vi "HapticSPM_write_virtual_only.vi"() -> ()   [LabVIEW 2022 SP3]
uses:
  Haptic-Programming-Interface/LabVIEW VIs/Haptic Prog Interface/Haptic Prog Interface.lvlib
panel:
  out "Value":dbl caption="Numeric" format="%#_2p"
  in  "Stop":bool
  out "Force vs Signal":cluster{dbl[], dbl[]}(graph)
  out "Signal & Force (Scaled)":dbl[][](graph)
  in  "Suggested Settings":bool=TRUE
  out "?":bool=TRUE
  out "Surface":dbl caption="Numeric" format="%#_2p"
  out "Z-Position":dbl caption="Numeric" format="%#_2p"
  out "y":string
  out "x":string
  out "scan data":dbl[][](array[numeric])
  out "2D Picture":picture
  out "Force":dbl(slide) scale=-3.0..3.0
  out "Frame String":string
  out "Reframed Position (m)":cluster{"x (m)":dbl, "y (m)":dbl, "z (m)":dbl} {"z (m)" format="%.1p"; "y (m)" format="%.1p"; "x (m)" format="%.1p"}
  out "Frame Properties (m)":T1
  in  "Function":string(combo)="0" caption="Combo Box"
  in  "Gain (mm/pm)":dbl=1.0 caption="Numeric" format="%.1g"
  in  "k":dbl=1.0 caption="Numeric" step=0.1 format="%.1g"
  in  "Setpoint":dbl=1e-10 caption="Numeric" step=1e-11 format="%.0p"
  in  "Gain":dbl=1.0 caption="Numeric" format="%.1g"
  out "Click Number":dbl caption="Numeric" format="%#_1g"
  in  "Planing Toggle":bool
  in  "Planing Reset":bool
  in  "Save":bool
  # "Super Ultra Mega Haptic SPM Controller 3000"
  # "Scan Window"
  # "Height"
  # "Signal"
  # "Force"
  # "Force"
  # "Planing"
  # "Surface Scale"
  # "Move pens in all three dimensions to calibrate\nClick \"enter\" to turn off recommended settings"
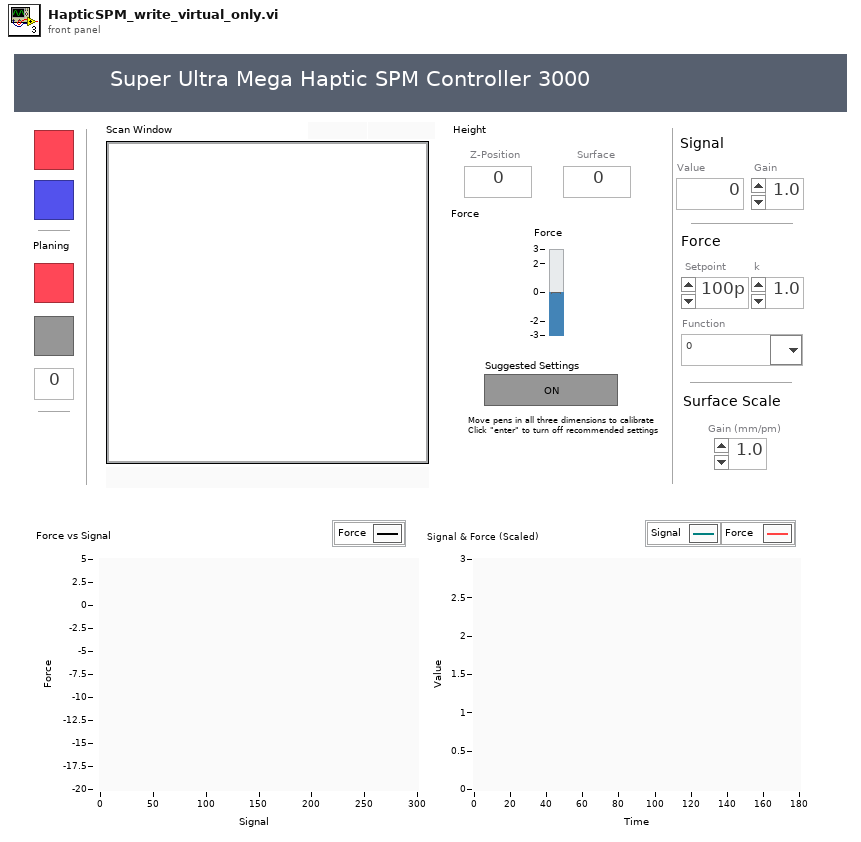
[diagram p1: front panel]
types:
  T1 = cluster{"Center coordinates (m)":cluster{"Xc":sgl, "Yc":sgl}, "Size (m)":cluster{"Width":sgl, "Height":sgl}}
  T2 = cluster{"Fx (N)":dbl, "Fy (N)":dbl, "Fz (N)":dbl}
  T3 = cluster{"kx (N/m)":dbl, "ky (N/m)":dbl, "kz (N/m)":dbl}
  T4 = cluster{"X Drag":bool, "Y Drag":bool, "Z Drag":bool}
  T5 = cluster{"Origin (m)":cluster{"X Origin (m)":dbl, "Y Origin (m)":dbl}, "Frame Size (m)":cluster{"FW (m)":dbl, "FH (m)":dbl}}
  T6 = cluster{"x (mm)":dbl, "y (mm)":dbl, "z (mm)":dbl}
  T7 = typedef "LVBoundsTypeDef.ctl" = cluster{"Width":u32, "Height":u32}
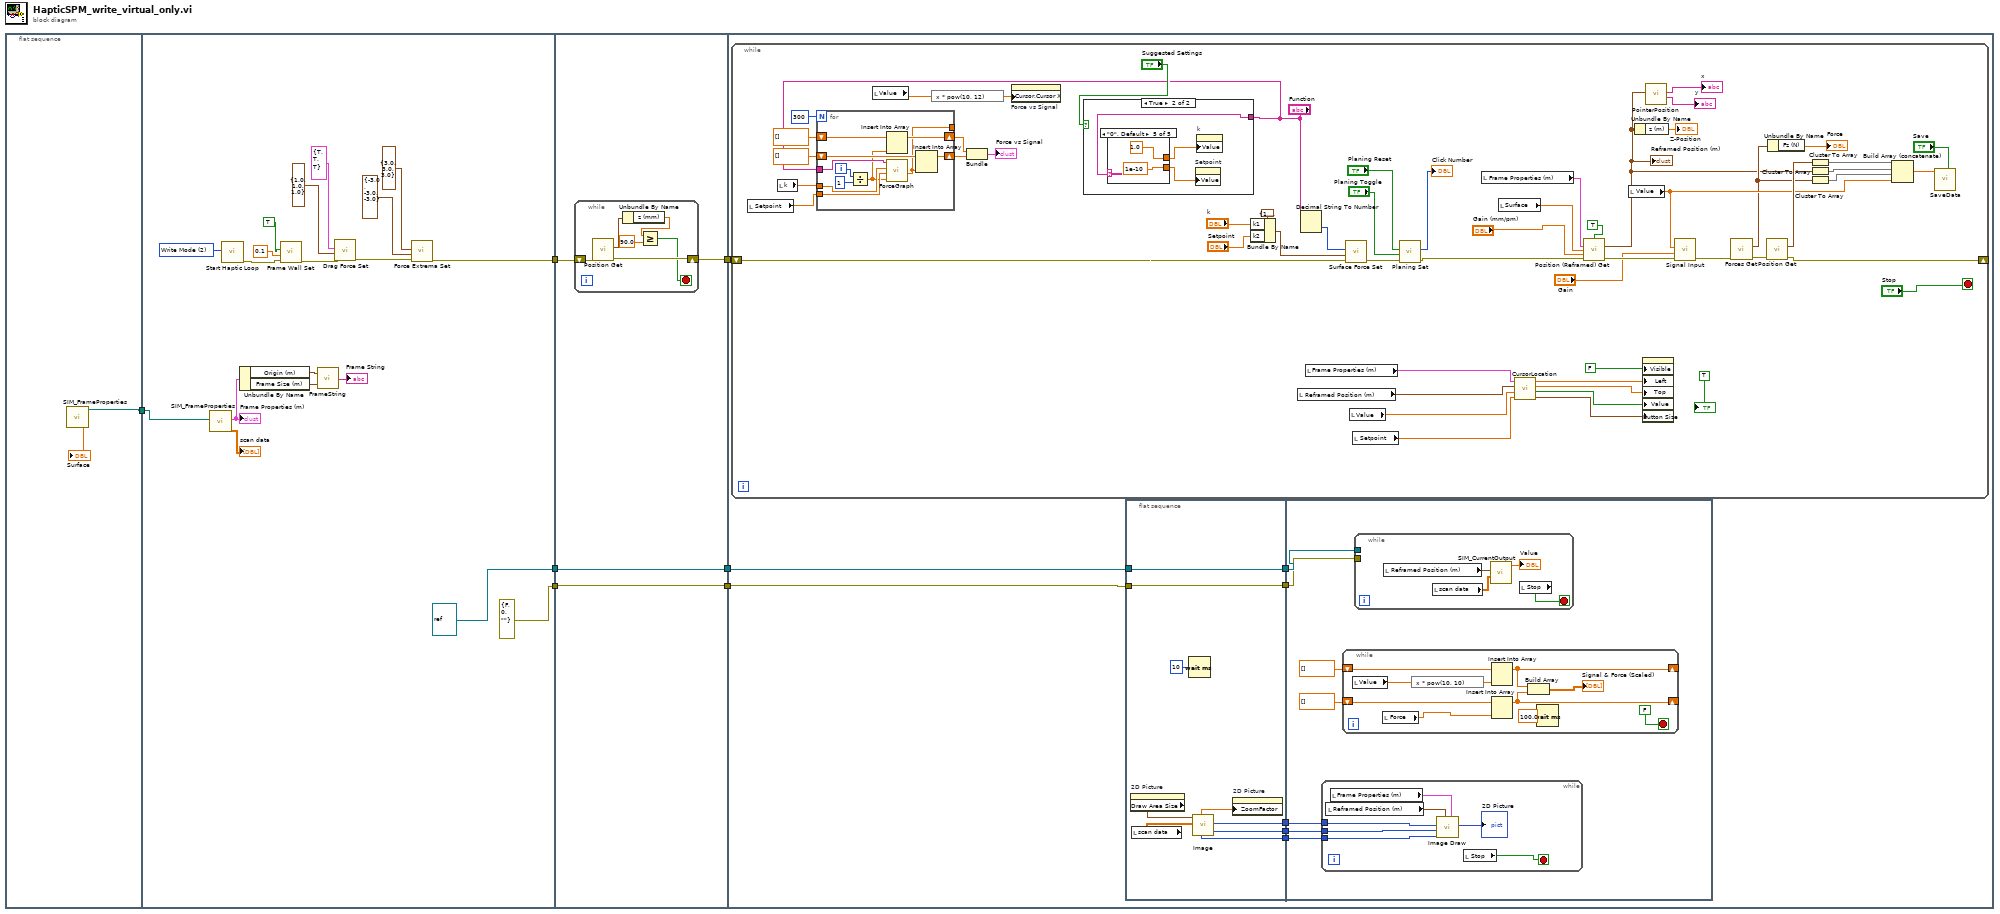
[diagram p0: block diagram]
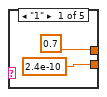
[diagram p3: hidden frame]
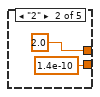
[diagram p4: hidden frame]
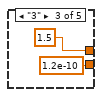
[diagram p5: hidden frame]
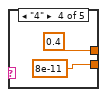
[diagram p6: hidden frame]
diagram:
  n1 = flat-sequence {
    tunnel: [w8] -> w1
    tunnel: [w26] -> w7
    tunnel: [refnum<vi> refnum ("Application ref out")] -> w4
    tunnel: [errorcluster {"status"=FALSE, "code"=0, "source"=""} ("error out")] -> w2
    tunnel: w1 -> [w14]
    tunnel: w7 -> [w32]
    tunnel: [w31] -> w6
    tunnel: [w30] -> w5
    tunnel: w4 -> [w30]
    tunnel: [w29] -> w3
    tunnel: w2 -> [w29]
    tunnel: w6 -> [w46]
    tunnel: w5 -> [w44]
    tunnel: w3 -> [w42]
    frame #0 {
      n2 = call "SIM_FrameProperties.vi"() -> ("Surf Loc (m)"=→"Surface":dbl, "new file path (Not A Path if cancelled)"=w8:path)  [unwired: 8 in, 2 out]
    }
    frame #1 {
      w28 = u16 2 items=["Custom Mode", "Read Mode", "Write Mode"] ("Mode Selection")
      n3 = call "SIM_FrameProperties.vi"("file path (dialog if empty)"=w14) -> ("data"=→"scan data":dbl[][], "Frame Properties (m)"=w12:T5)  [unwired: 7 in, 2 out]
      "Frame Properties (m)" <- w12
      n4 = call <userlib>:"Start Haptic Loop.vi"("Mode Selection"=w28) -> ("error out"=w19:errorcluster)  [unwired: 10 in]
      n5 = Unbundle By Name(w12) -> ("Origin (m)"=w15:cluster{"X Origin (m)":dbl, "Y Origin (m)":dbl}, "Frame Size (m)"=w16:cluster{"FW (m)":dbl, "FH (m)":dbl})
      n6 = call <userlib>:"Frame Wall Set.vi"("error in (no error)"=w19, "Wall Stiffness (N/m)"=0.1 ("Wall Stiffness"), "Restrict to Frame"=TRUE) -> ("error out"=w18:errorcluster)  [unwired: 8 in]
      n7 = call "FrameString.vi"("Size (m)"=w16, "Center coordinates (m)"=w15) -> ("string"=→"Frame String":string)
      n8 = call <userlib>:"Drag Force Set.vi"("error in (no error)"=w18, "Drag Coefficients (N/m)"=T3 {"kx (N/m)"=1.0, "ky (N/m)"=1.0, "kz (N/m)"=1.0} ("Drag Coefficients"), "Drag Force Toggles"=T4 {"X Drag"=TRUE, "Y Drag"=TRUE, "Z Drag"=TRUE}) -> ("error out"=w27:errorcluster)  [unwired: 8 in]
      n9 = call <userlib>:"Force Extrema Set.vi"("error in (no error)"=w27, "Minimum Force (N)"=T2 {"Fx (N)"=-3.0, "Fy (N)"=-3.0, "Fz (N)"=-3.0} ("Minimum Force"), "Maximum Force (N)"=T2 {"Fx (N)"=3.0, "Fy (N)"=3.0, "Fz (N)"=3.0} ("Maximum Force")) -> ("error out"=w26:errorcluster)  [unwired: 8 in]
    }
    frame #2 {
      n10 = while {
        shift-right: [w37] -> w31
        shift-left: w32 -> [w38]
        stop <- w33 stop-if-true
        n11 = call <userlib>:"Position Get.vi"("error in (no error)"=w38) -> ("error out"=w37:errorcluster, "Position"=w36:T6)  [unwired: 9 in]
        n12 = Unbundle By Name(w36) -> ("z (mm)"=w35:dbl)
        n13 = Greater Or Equal?(x=w35, y=90.0) -> (x >= y?=w33:bool)
      }
    }
    frame #3 {
      n14 = while {
        shift-right: [w133] -> _
        shift-left: w46 -> [w139]
        stop <- "Stop" stop-if-true
        n15 = local read "Setpoint"() -> (w85:dbl)
        n16 = local read "k"() -> (w86:dbl)
        n17 = for {
          N: 300 -> [_]
          shift-right: [w150] -> w94
          shift-left: dbl[] [] -> [w148]
          shift-right: [w149] -> w95
          shift-left: dbl[] [] -> [w147]
          tunnel: "Function" -> [w143]
          tunnel: [w146] -> _
          tunnel: w85 -> [w145]
          tunnel: w86 -> [w144]
          i -> [w141]
          n18 = Divide(x=w141, y=1) -> (x/y=w140:dbl)
          n19 = Insert Into Array(array=w147, new element=w140) -> (w149:dbl[])  [unwired: 1 in]
          n20 = call "ForceGraph.vi"("number"=w140, "Setpoint"=w145, "k"=w144, "Function"=w143) -> ("force"=w146:dbl)  [unwired: 7 in]
          n21 = Insert Into Array(array=w148, new element=w146) -> (w150:dbl[])  [unwired: 1 in]
        }
        n22 = local read "Value"() -> (w87:dbl)
        n23 = expression code="x * pow(10, 12)"(w87) -> (w90:dbl)
        n24 = Bundle(w95, w94) -> (→"Force vs Signal":cluster{dbl[], dbl[]})  [unwired: 1 in]
        n25 = property on="Force vs Signal" class="XYGraph (strict)"("Cursor.Cursor X"=w90) -> ()  [unwired: 2 in, 2 out]
        n26 = case shown="True" "Suggested Settings" {
          tunnel: "Function" -> [_ w153]
          frame False {
          }
          frame True {
            n27 = case shown="\"0\", Default" w153 {
              tunnel: [0.7 2.0 1.5 0.4 1.0] -> w152
              tunnel: [2.4e-10 1.4e-10 1.2e-10 8e-11 1e-10] -> w151
              frame "1" {
              }
              frame "2" {
              }
              frame "3" {
              }
              frame "4" {
              }
              frame "0", Default {
              }
            }
            n28 = property on="Setpoint" class="DigNum (strict)"("Value"=w151) -> ()  [unwired: 2 in, 2 out]
            n29 = property on="k" class="DigNum (strict)"("Value"=w152) -> ()  [unwired: 2 in, 2 out]
          }
        }
        n30 = Bundle By Name(cluster=cluster{"k1":dbl, "k2":dbl, "k3":dbl, "k4":dbl} {"k1"=1.0, "k2"=1.0, "k3"=1.0, "k4"=1.0} ("Force Constants"), "k1"="k", "k2"="Setpoint") -> (w126:cluster{"k1":dbl, "k2":dbl, "k3":dbl, "k4":dbl})
        n31 = local read "Reframed Position (m)"() -> (w98:cluster{"x (m)":dbl, "y (m)":dbl, "z (m)":dbl})
        n32 = Decimal String To Number(string="Function") -> (number=w123:i32)  [unwired: 2 in, 1 out]
        n33 = local read "Frame Properties (m)"() -> (w102:T1)
        n34 = call <userlib>:"Surface Force Set.vi"("error in (no error)"=w139, "Force Constants"=w126, "Force Settings"=w123) -> ("error out"=w138:errorcluster)  [unwired: 8 in]
        n35 = local read "Value"() -> (w101:dbl)
        n36 = local read "Setpoint"() -> (w100:dbl)
        n37 = call <userlib>:"Planing Set.vi"("error in (no error)"=w138, "Planing"="Planing Toggle", "Reset"="Planing Reset") -> ("error out"=w129:errorcluster, "Number of Clicks"=→"Click Number":i8)  [unwired: 7 in]
        n38 = local read "Frame Properties (m)"() -> (w113:T1)
        n39 = local read "Surface"() -> (w137:dbl)
        n40 = call "CursorLocation.vi"("Setpoint"=w100, "Value"=w101, "Position (Reframed)"=w98, "Frame Properties (m)"=w102) -> ("Cursor Size"=w103:cluster{"Width":i32, "Height":i32}, "Current Above Setpoint?"=w104:bool, "Y-Coordinate"=w105:dbl, "X-Coordinate"=w106:dbl)
        n41 = call <userlib>:"Position (Reframed) Get.vi"("Z Rescaling"=TRUE, "Frame Properties (m)"=w113, "Surface Location (m)"=w137, "Scaling (mm per pm)"="Gain (mm/pm)", "error in (no error)"=w129) -> ("Reframed Position (m)"=w109:cluster{"x (m)":dbl, "y (m)":dbl, "z (m)":dbl}, "error out"=w135:errorcluster)  [unwired: 9 in]
        "Reframed Position (m)" <- w109
        n42 = local read "Value"() -> (w117:dbl)
        n43 = Unbundle By Name(w109) -> ("z (m)"=→"Z-Position":dbl)
        n44 = property class="Bool (strict)"("Visible"=FALSE, "Left"=w106, "Top"=w105, "Value"=w104, "Button Size"=w103) -> ()  [unwired: 2 in, 2 out]
        n45 = call "PointerPosition.vi"("Reframed Position (m)"=w109) -> ("y string"=→"y":string, "x string"=→"x":string)  [unwired: 9 in]
        n46 = call <userlib>:"Signal Input.vi"("error in (no error)"=w135, "Gain"="Gain", "Signal"=w117) -> ("error out"=w136:errorcluster)  [unwired: 8 in]
        n47 = call <userlib>:"Forces Get.vi"("error in (no error)"=w136) -> ("error out"=w134:errorcluster, "Force (N)"=w114:T2)  [unwired: 9 in]
        n48 = call <userlib>:"Position Get.vi"("error in (no error)"=w134) -> ("error out"=w133:errorcluster, "Position"=w121:T6)  [unwired: 9 in]
        n49 = Unbundle By Name(w114) -> ("Fz (N)"=→"Force":dbl)
        n50 = Cluster To Array(cluster=w121) -> (array=w120:dbl[])
        n51 = Cluster To Array(cluster=w109) -> (array=w119:dbl[])
        n52 = Cluster To Array(cluster=w114) -> (array=w118:dbl[])
        n53 = Build Array (concatenate)(w120, w119, w118, w117) -> (w116:dbl[])
        n54 = call "SaveData.vi"("Save"="Save", "Data"=w116) -> ()  [unwired: 10 in]
        "?" <- TRUE
      }
      n55 = flat-sequence {
        tunnel: [w54] -> w45
        tunnel: w44 -> [w54]
        tunnel: [w53] -> w43
        tunnel: w42 -> [w53]
        tunnel: [w49] -> w41
        tunnel: [w48] -> w40
        tunnel: [w47] -> w39
        tunnel: w45 -> [w57]
        tunnel: w43 -> [w56]
        tunnel: w41 -> [w62]
        tunnel: w40 -> [w61]
        tunnel: w39 -> [w60]
        frame #0 {
          n56 = property on="2D Picture" class="Pict"() -> ("Draw Area Size"=w52:T7)  [unwired: 2 in, 2 out]
          n57 = local read "scan data"() -> (w50:dbl[][])
          n58 = Wait (ms)(milliseconds to wait=u32 10) -> ()  [unwired: 1 out]
          n59 = call "Image.vi"("data"=w50, "Draw Area Size"=w52) -> ("Rectangle.bottom"=w47:i16, "Rectangle.right"=w48:i16, "new picture"=w49:picture, "ZoomFactor"=w51:dbl)  [unwired: 6 in]
          n60 = property on="2D Picture" class="Pict"("ZoomFactor"=w51) -> ()  [unwired: 2 in, 2 out]
        }
        frame #1 {
          n61 = while {
            tunnel: w62 -> [w82]
            tunnel: w61 -> [w81]
            tunnel: w60 -> [w80]
            stop <- w83 stop-if-true
            n62 = local read "Reframed Position (m)"() -> (w79:cluster{"x (m)":dbl, "y (m)":dbl, "z (m)":dbl})
            n63 = local read "Frame Properties (m)"() -> (w78:T1)
            n64 = call "Image Draw.vi"("Frame Properties (m)"=w78, "Reframed Position (m)"=w79, "ih"=w80, "iw"=w81, "picture"=w82) -> ("new picture"=→"2D Picture":picture)  [unwired: 6 in]
            n65 = local read "Stop"() -> (w83:bool)
          }
          n66 = while {
            shift-right: [w71] -> _
            shift-left: dbl[] [] ("element") -> [w70]
            shift-right: [w72] -> _
            shift-left: dbl[] [] -> [w73]
            stop <- FALSE stop-if-true
            n67 = local read "Value"() -> (w68:dbl)
            n68 = local read "Force"() -> (w67:dbl)
            n69 = expression code="x * pow(10, 10)"(w68) -> (w74:dbl)
            n70 = Insert Into Array(array=w70, new element=w74) -> (w71:dbl[])  [unwired: 1 in]
            n71 = Insert Into Array(array=w73, new element=w67) -> (w72:dbl[])  [unwired: 1 in]
            n72 = Build Array(w71, w72) -> (→"Signal & Force (Scaled)":dbl[][])
            n73 = Wait (ms)(milliseconds to wait=100.0) -> ()  [unwired: 1 out]
          }
          n74 = while {
            tunnel: w57 -> [_]
            tunnel: w56 -> [_]
            stop <- w65 stop-if-true
            n75 = local read "Reframed Position (m)"() -> (w66:cluster{"x (m)":dbl, "y (m)":dbl, "z (m)":dbl})
            n76 = local read "scan data"() -> (w64:dbl[][])
            n77 = call "SIM_CurrentOutput.vi"("array"=w64, "Position (Reframed)"=w66) -> ("Current Out (A)"=→"Value":dbl)  [unwired: 8 in, 1 out]
            n78 = local read "Stop"() -> (w65:bool)
          }
        }
      }
    }
  }
